vi "trapezoidal_v1.vi"(6 "number of cycles":dbl=2.0, 8 "phase":dbl format="%.2p", 9 "frequency":dbl=1.0 format="%#_13g", 10 "Offset in":dbl, 11 "Amplitude in":dbl) -> (3 "Waveform Graph":waveform(dbl)(graph))   [LabVIEW 2020]
uses:
  <vilib>/measure/NI_MABase.lvlib
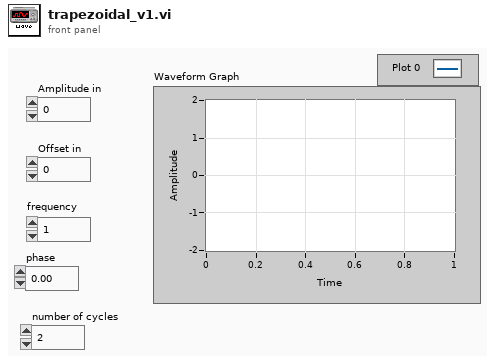
[diagram p1: front panel]
types:
  T1 = enum16{"Sine Wave", "Triangle Wave", "Square Wave", "Sawtooth Wave"}
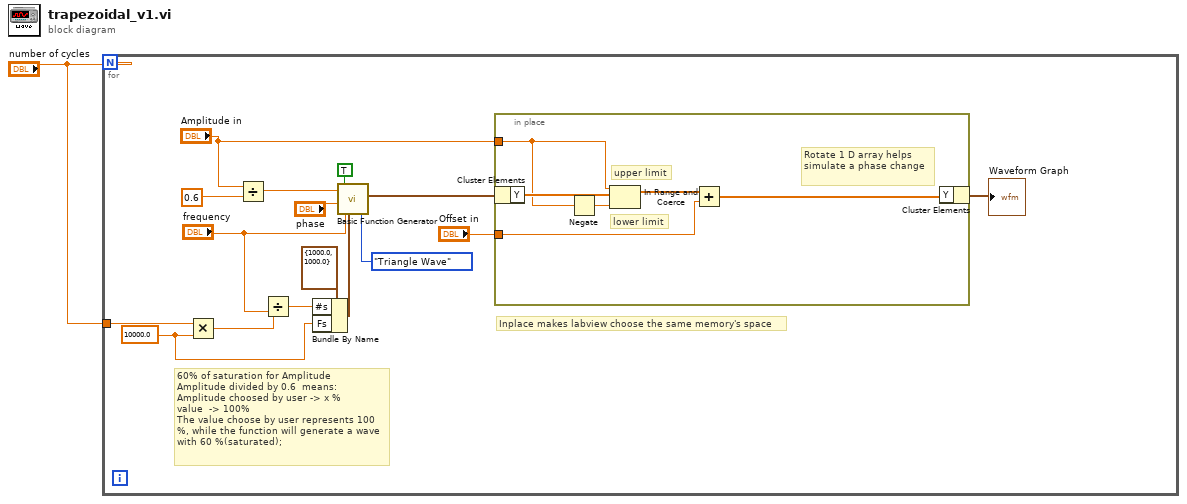
[diagram p0: block diagram]
diagram:
  n1 = for {
    N: "number of cycles" -> [_]
    tunnel: "number of cycles" -> [w6]
    w3 = 10000.0 ("y")
    # "Inplace makes labview choose the same memory's space"
    # "60% of saturation for Amplitude\nAmplitude divided by 0.6  means:\nAmplitude choosed by user -> x %\nvalue  -> 100%\nThe value choose by user represents 100 %, while the function will generate a wave with 60 %(saturated);"
    n2 = Multiply(x=w6, y=w3) -> (x*y=w7:dbl)
    n3 = Divide(x="Amplitude in", y=0.6 ("x")) -> (x/y=w12:dbl)
    n4 = Divide(x=w7, y="frequency") -> (x/y=w4:dbl)
    n5 = Bundle By Name(cluster=cluster{"Fs":dbl, "#s":dbl} {"Fs"=1000.0, "#s"=1000.0} ("sampling info"), "#s"=w4, "Fs"=w3) -> (w8:cluster{"Fs":dbl, "#s":dbl})
    n6 = call <vilib>:"Basic Function Generator.vi"("reset signal"=TRUE, "sampling info"=w8, "signal type"=T1."Triangle Wave", "phase"="phase", "amplitude"=w12, "frequency"="frequency") -> ("signal out"=w16:waveform(dbl))  [unwired: 3 in, 2 out]
    n7 = in-place {
      in-place-border: "Amplitude in" -> [w21]
      in-place-border: "Offset in" -> [w19]
      # "Rotate 1 D array helps simulate a phase change"
      # "lower limit"
      # "upper limit"
      n8 = in-place-cluster #1(w16) -> ("Y"=w23:dbl[])
      n9 = Negate(x=w21) -> (-x=w22:dbl)
      n10 = In Range and Coerce(upper limit=w21, x=w23, lower limit=w22) -> (coerced(x)=w20:dbl[])  [unwired: 1 out]
      n11 = Add(x=w20, y=w19) -> (x+y=w18:dbl[])
      n12 = in-place-cluster #1("Y"=w18) -> (→"Waveform Graph":waveform(dbl))
    }
  }
